vi "add_paths_to_bin.vi"(8 "error in (no error)":errorcluster, 10 "Files to transfer in":path[](array[path]), 11 "Files to transfer bin file":refnum<file>) -> (0 "error out":errorcluster, 2 "Files to transfer out":path[](array[path]), 3 "path out":path)   [LabVIEW 2017, in "labview-standard-library.lvlib"]
uses:
  labview-standard-library.lvlib
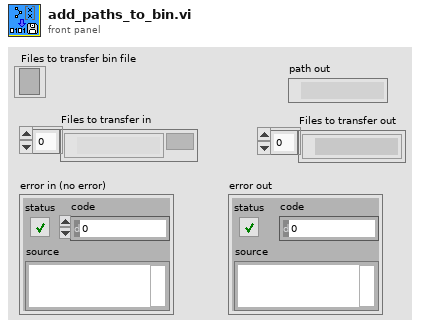
[diagram p1: front panel]
types:
  T1 = enum16{"big-endian, network order", "native, host order", "little-endian"}
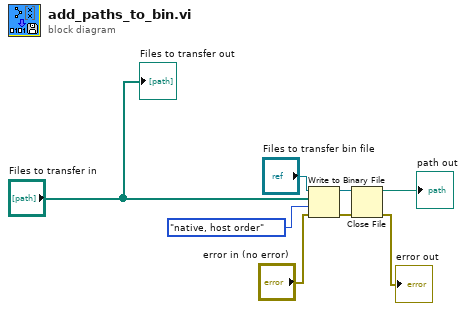
[diagram p0: block diagram]
diagram:
  n1 = Write to Binary File(file (use dialog)="Files to transfer bin file", data="Files to transfer in", error in="error in (no error)", 9:T1."native, host order" ("byte order (0:big-endian, network order)")) -> (refnum out=w6:refnum<file>, error out=w5:errorcluster)  [unwired: 2 in, 1 out]
  n2 = Close File(refnum=w6, error in=w5) -> (path=→"path out":path, error out=→"error out":errorcluster)
  "Files to transfer out" <- "Files to transfer in"
